vi "Starter Kit 2.0 Host Controller.vi"() -> ()   [LabVIEW 2010]
doc: "This VI runs on a desktop where it remotely controls the Starter Kit robot through a TCP connection. Run the robot receiver VI on the RT target before running this VI."
uses:
  Support VIs/Motor Velocity.ctl
  Support VIs/Starter Kit Message.ctl
  <vilib>/robotics/Steering/Steering Frame/Apply Steering Frame Velocity to Motors.vi
  <vilib>/robotics/Starter Kit/2.0/NI_Robotics_Starter Kit Host_2.0.lvlib
  <vilib>/robotics/Steering/Steering Frame/NI_Robotics_Steering Frame.lvclass
panel:
  in  "Servo Angle (rad)":dbl(slide) scale=1.0..-1.0
  in  "Port (12345)":u16=12345
  in  "Robot IP Address":string="0.0.0.0"
  in  "stop":bool
  in  "Angular Velocity (rad/s)":dbl(slide) scale=2.0..-2.0
  in  "Forward Velocity (m/s)":dbl(slide) scale=-0.5..0.5
  # "Set Robot IP Address before running this VI."
  # "Move the Forward Velocity slider to control the forward velocity component of the robot.\n\nMove the Angular Velocity slider to control the counterclockwise rotation of the robot.\n\nMove the Servo Angle slider to control the counterclockwise angle of the ultrasonic sensor on the robot.  This example does not collect range data from the sensor."
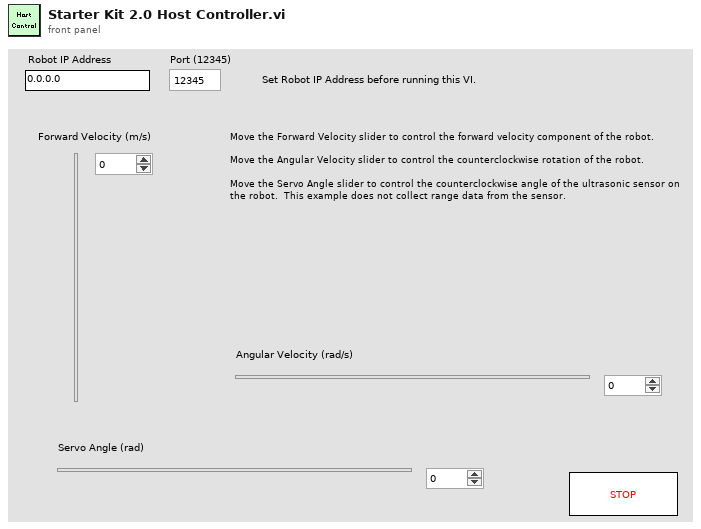
[diagram p1: front panel]
types:
  T1 = enum16{"Heartbeat", "Motor Vel SP", "Servo Angle", "Stop"}
  T2 = typedef "Starter Kit Message.ctl" = cluster{"message type":enum16{"Heartbeat", "Motor Vel SP", "Servo Angle", "Stop"}, "message data":variant}
  T3 = typedef "Motor Velocity.ctl" = cluster{"left motor ccw vel":dbl, "right motor ccw vel":dbl}
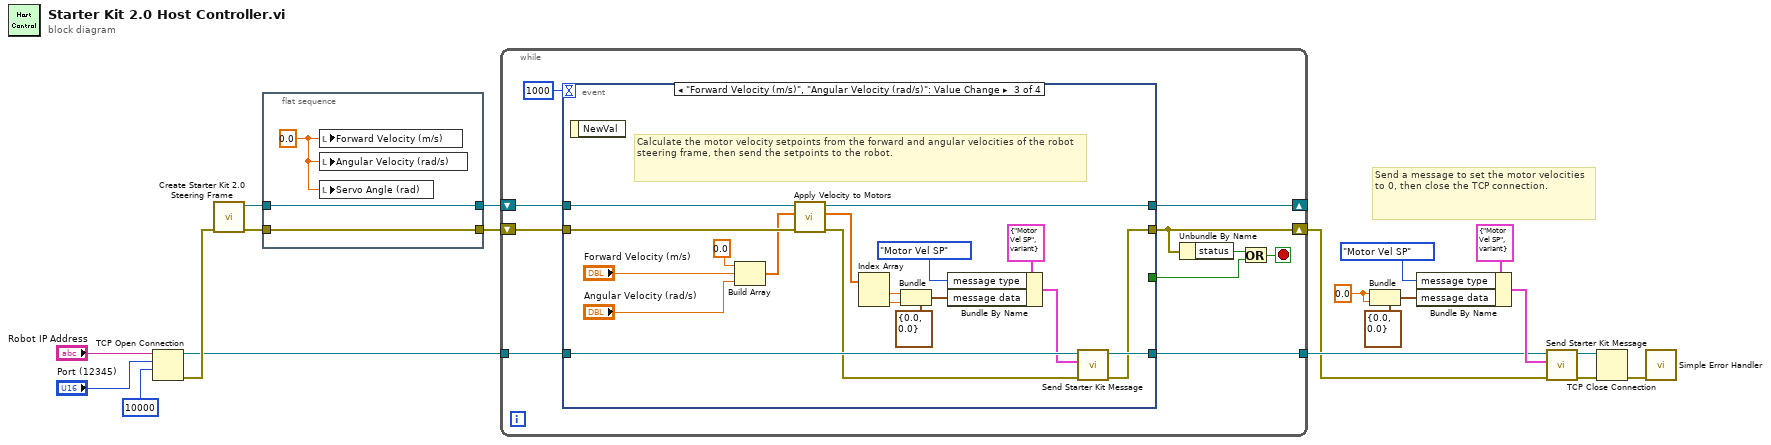
[diagram p0: block diagram]
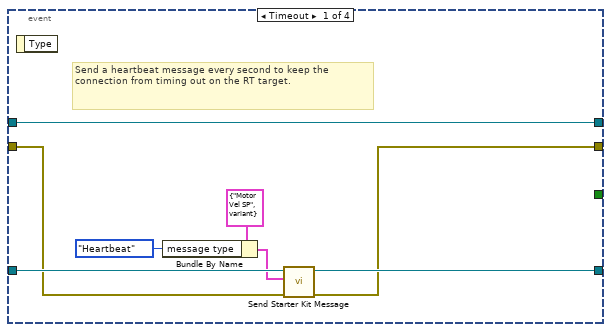
[diagram p2: hidden frame]
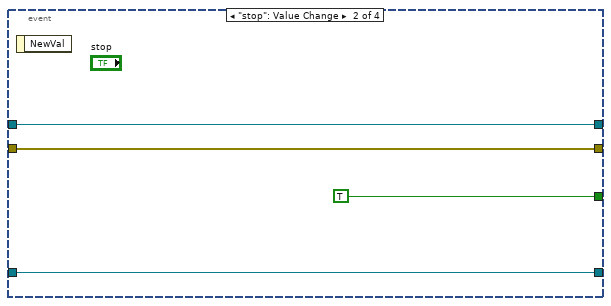
[diagram p3: hidden frame]
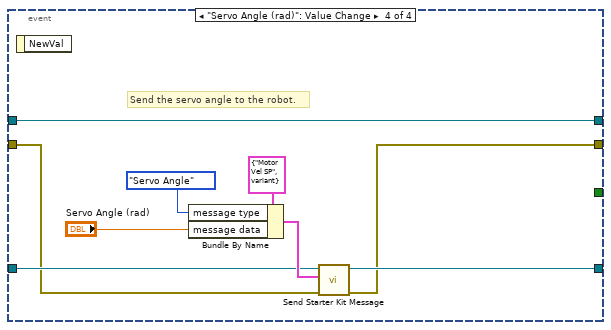
[diagram p4: hidden frame]
diagram:
  w9 = 0.0 ("left motor ccw vel")
  # "Send a message to set the motor velocities to 0, then close the TCP connection."
  n1 = TCP Open Connection(address="Robot IP Address", remote port or service name="Port (12345)", timeout ms (60000)=10000) -> (connection ID=w17:refnum<k5>, error out=w18:errorcluster)  [unwired: 1 in, 1 out]
  n2 = call <vilib>:"Create Starter Kit 2.0 Steering Frame.vi"("error in (no error)"=w18) -> ("error out"=w4:errorcluster, "starter kit differential steering frame"=w3:refnum<class "NI_Robotics_Differential Steering Frame.lvclass">)  [unwired: 9 in]
  n3 = flat-sequence {
    tunnel: w4 -> [w23]
    tunnel: w3 -> [w22]
    tunnel: [w23] -> w2
    tunnel: [w22] -> w1
    frame #0 {
      w21 = 0.0 ("Forward Velocity (m/s)")
      n4 = local write "Forward Velocity (m/s)"(w21) -> ()
      n5 = local write "Angular Velocity (rad/s)"(w21) -> ()
      n6 = local write "Servo Angle (rad)"(w21) -> ()
    }
  }
  n7 = while {
    tunnel: w17 -> [w32]
    shift-right: [w29] -> _
    shift-left: w1 -> [w31]
    shift-right: [w27] -> w10
    shift-left: w2 -> [w30]
    tunnel: [w28] -> w11
    stop <- w25 stop-if-true
    n8 = event shown="[2] \"Forward Velocity (m/s)\", \"Angular Velocity (rad/s)\": Value Change" {
      selector: _ -> [_ _ _ _]
      dyn-events: _ -> [_ _ _ _]
      timeout: 1000 -> [_ _ _ _]
      tunnel: [_ TRUE _ _] -> w24
      tunnel: w32 -> [w39 w43 w51 w69]
      tunnel: w31 -> [w41 w44 w64 w73]
      tunnel: w30 -> [w35 w42 w62 w67]
      tunnel: [w41 w44 w63 w73] -> w29
      tunnel: [w34 w42 w47 w66] -> w27
      tunnel: [w38 w43 w50 w68] -> w28
      event Timeout {
        # "Send a heartbeat message every second to keep the connection from timing out on the RT target."
        n9 = event-data() -> ()  [unwired: 1 in, 1 out]
        n10 = Bundle By Name(cluster=T2 {"message type"=enum."Motor Vel SP", "message data"=variant} ("message"), "message type"=T1."Heartbeat") -> (w37:T2)
        n11 = call "Send Starter Kit Message.vi"("error in (no error)"=w35, "message"=w37, "connection ID in"=w39) -> ("error out"=w34:errorcluster, "connection ID out"=w38:refnum<k5>)  [unwired: 7 in]
      }
      event "stop": Value Change {
        n12 = event-data() -> ()  [unwired: 1 in, 1 out]
      }
      event "Forward Velocity (m/s)", "Angular Velocity (rad/s)": Value Change {
        # "Calculate the motor velocity setpoints from the forward and angular velocities of the robot steering frame, then send the setpoints to the robot."
        n13 = event-data() -> ()  [unwired: 1 in, 1 out]
        n14 = Build Array(0.0 ("element"), "Forward Velocity (m/s)", "Angular Velocity (rad/s)") -> (w58:dbl[])
        n15 = call-poly <vilib>:"Apply Velocity to Motors.vi"("error in (no error)"=w62, "steering frame velocity"=w58, "steering frame in"=w64) -> ("error out"=w48:errorcluster, "ccw motor velocity setpoints"=w57:dbl[], "steering frame out"=w63:refnum<class "NI_Robotics_Differential Steering Frame.lvclass">)  [unwired: 4 in, 2 out]
        n16 = Index Array(array=w57) -> (element #1=w55:dbl, element #2=w56:dbl)  [unwired: 2 in]
        n17 = Bundle(cluster=T3 {"left motor ccw vel"=0.0, "right motor ccw vel"=0.0} ("motor velocity"), "left motor ccw vel"=w55, "right motor ccw vel"=w56) -> (w52:T3)
        n18 = Bundle By Name(cluster=T2 {"message type"=enum."Motor Vel SP", "message data"=variant} ("message"), "message type"=T1."Motor Vel SP", "message data"=w52) -> (w49:T2)
        n19 = call "Send Starter Kit Message.vi"("error in (no error)"=w48, "message"=w49, "connection ID in"=w51) -> ("error out"=w47:errorcluster, "connection ID out"=w50:refnum<k5>)  [unwired: 7 in]
      }
      event "Servo Angle (rad)": Value Change {
        # "Send the servo angle to the robot."
        n20 = event-data() -> ()  [unwired: 1 in, 1 out]
        n21 = Bundle By Name(cluster=T2 {"message type"=enum."Motor Vel SP", "message data"=variant} ("message"), "message type"=T1."Servo Angle", "message data"="Servo Angle (rad)") -> (w71:T2)
        n22 = call "Send Starter Kit Message.vi"("error in (no error)"=w67, "message"=w71, "connection ID in"=w69) -> ("error out"=w66:errorcluster, "connection ID out"=w68:refnum<k5>)  [unwired: 7 in]
      }
    }
    n23 = Unbundle By Name(w27) -> ("status"=w26:bool)
    n24 = Or(x=w26, y=w24) -> (x .or. y?=w25:bool)
  }
  n25 = Bundle(cluster=T3 {"left motor ccw vel"=0.0, "right motor ccw vel"=0.0} ("motor velocity"), "left motor ccw vel"=w9, "right motor ccw vel"=w9) -> (w14:T3)
  n26 = Bundle By Name(cluster=T2 {"message type"=enum."Motor Vel SP", "message data"=variant} ("message"), "message type"=T1."Motor Vel SP", "message data"=w14) -> (w15:T2)
  n27 = call "Send Starter Kit Message.vi"("error in (no error)"=w10, "message"=w15, "connection ID in"=w11) -> ("error out"=w7:errorcluster, "connection ID out"=w6:refnum<k5>)  [unwired: 7 in]
  n28 = TCP Close Connection(connection ID=w6, error in (no error)=w7) -> (error out=w5:errorcluster)  [unwired: 1 in, 1 out]
  n29 = call <vilib>:"Simple Error Handler.vi"("error in (no error)"=w5) -> ()  [unwired: 1 in, 8 out]
